vi "Biquadratic peak fit gradient ascent optimisation.vi"(4 "tol^2":dbl=1e-09 format="%#_13g", 5 "Grad step":dbl=0.01 format="%#_13g", 6 "Max iters":i32=10000, 7 "3x3 peak patch":dbl[][](array[numeric])) -> (0 "Iterations":i32, 1 "Sub-pixel convergence":bool, 2 "dy":dbl, 3 "dx":dbl)   [LabVIEW 2015]
uses:
  <vilib>/Analysis/Matrix/Datatypes/RealMatrix.ctl
  <vilib>/Analysis/baseanly.llb/A x Vector.vi
  <vilib>/Analysis/Matrix/NI_Matrix.lvlib
  <vilib>/Analysis/NI_AALBase.lvlib
panel:
  # "Paul Nathan 09/06/2015,\n22/03/2016 (step size limit)"
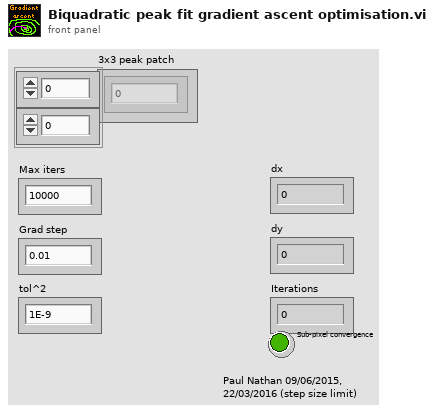
[diagram p1: front panel]
types:
  T1 = typedef "NI_Matrix.lvlib/RealMatrix.ctl" = dbl[][]
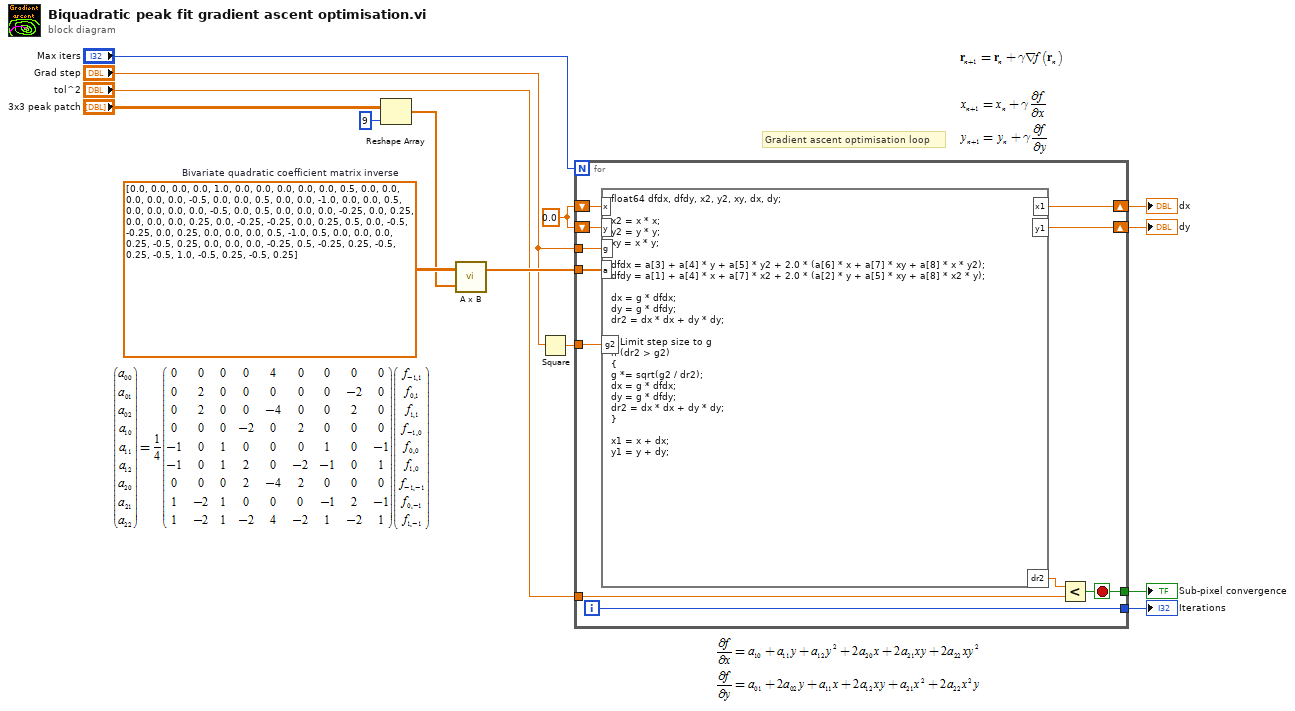
[diagram p0: block diagram]
diagram:
  w11 = 0.0
  w13 = T1 [[0.0, 0.0, 0.0, 0.0, 1.0, 0.0, 0.0, 0.0, 0.0], [0.0, 0.5, 0.0, 0.0, 0.0, 0.0, 0.0, -0.5, 0.0], [0.0, 0.5, 0.0, 0.0, -1.0, 0.0, 0.0, 0.5, 0.0], [0.0, 0.0, 0.0, -0.5, 0.0, 0.5, 0.0, 0.0, 0.0], [-0.25, 0.0, 0.25, 0.0, 0.0, 0.0, 0.25, 0.0, -0.25], [-0.25, 0.0, 0.25, 0.5, 0.0, -0.5, -0.25, 0.0, 0.25], [0.0, 0.0, 0.0, 0.5, -1.0, 0.5, 0.0, 0.0, 0.0], [0.25, -0.5, 0.25, 0.0, 0.0, 0.0, -0.25, 0.5, -0.25], [0.25, -0.5, 0.25, -0.5, 1.0, -0.5, 0.25, -0.5, 0.25]]  # Bivariate quadratic coefficient matrix inverse
  # "Gradient ascent optimisation loop"
  n1 = Reshape Array("3x3 peak patch", 9 ("dimension size")) -> (w12:dbl[])
  n2 = call-poly <vilib>:"A x B.vi"("Vector"=w12, "A"=w13) -> ("A x Vector"=w10:dbl[])  [unwired: 1 out]
  n3 = Square(x="Grad step") -> (x^2=w2:dbl)
  n4 = for {
    N: "Max iters" -> [_]
    shift-right: [w21] -> w5
    shift-left: w11 -> [w22]
    shift-right: [w20] -> w4
    shift-left: w11 -> [w23]
    tunnel: "Grad step" -> [w24]
    tunnel: w10 -> [w25]
    tunnel: "tol^2" -> [w18]
    tunnel: [w17] -> w9
    tunnel: [w16] -> w7
    tunnel: w2 -> [w15]
    i -> [w17]
    stop <- w16 stop-if-true
    n5 = formula code="float64 dfdx, dfdy, x2, y2, xy, dx, dy;\n\nx2 = x * x;\ny2 = y * y;\nxy = x * y;\n\ndfdx = a[3] + a[4] * y + a[5] * y2 + 2.0 * (a[6] * x + a[7] * xy + a[8] * x * y2);\ndfdy = a[1] + a[4] * x + a[7] * x2 + 2.0 * (a[2] * y + a[5] * xy + a[8] * x2 * y);\n\ndx = g * dfdx;\ndy = g * dfdy;\ndr2 = dx * dx + dy * dy;\n\n// Limit step size to g\nif (dr2 > g2)\n{\ng *= sqrt(g2 / dr2);\ndx = g * dfdx;\ndy = g * dfdy;\ndr2 = dx * dx + dy * dy;\n}\n\nx1 = x + dx;\ny1 = y + dy;"("x"=w22, "y"=w23, "g"=w24, "a"=w25, "g2"=w15) -> ("x1"=w21:dbl, "y1"=w20:dbl, "dr2"=w19:dbl)
    n6 = Less?(x=w19, y=w18) -> (x < y?=w16:bool)
  }
  "Iterations" <- w9
  "Sub-pixel convergence" <- w7
  "dx" <- w5
  "dy" <- w4
